vi "GNSS RF Test Set Parameters.vi"(8 "error in (no error)":errorcluster, 10 "Parameters":T1={"GNSS Standard"=enum."GPS", "Frequency (Hz)"=0.0, "Auto Level"=FALSE, "Power (dBm)"=0.0, "External Attenuation (dB)"=0.0, "Measurement Interval (s)"=1000.0, "Pattern"=enum."PN9", "Enable Averaging"=FALSE, "Type Of Averaging"=enum."MEAN", "Number of Averages"=0, "Waveform Name"="", "Enable Traces"=FALSE} {"External Attenuation (dB)" format="%.1g"; "Power (dBm)" format="%.1g"}, 11 "Template Tx Test in":refnum<class "niDTS GNSS RF Test.lvclass">) -> (0 "error out":errorcluster, 3 "Template Tx Test out":refnum<class "niDTS GNSS RF Test.lvclass">)   [LabVIEW 2015, in "niDTS GNSS.lvlib" / "niDTS GNSS RF Test.lvclass"]
uses:
  niDTS GNSS RF Test.lvclass
  Includes/niDTS GNSS RF Test INC Parameters.ctl
  niDTS GNSS RF Test.lvclass/niDTS GNSS RF Test.ctl
  niDTS GNSS.lvlib
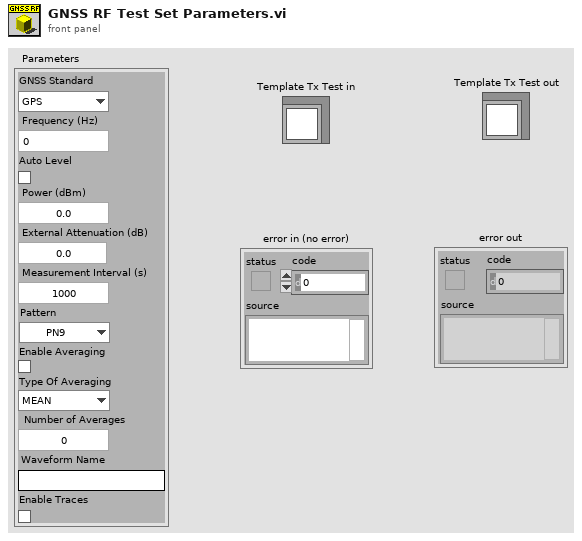
[diagram p1: front panel]
types:
  T1 = typedef "niDTS GNSS.lvlib/niDTS GNSS RF Test INC Parameters.ctl" = cluster{"GNSS Standard":enum16{"GPS", "GLONASS", "Galileo", "Beidou"}, "Frequency (Hz)":dbl, "Auto Level":bool, "Power (dBm)":dbl, "External Attenuation (dB)":dbl, "Measurement Interval (s)":dbl, "Pattern":enum16{"0", "1", "01", "00001111", "PN9"}, "Enable Averaging":bool, "Type Of Averaging":enum16{"MEAN", "MAX", "MIN", "MAXMIN"}, "Number of Averages":i32, "Waveform Name":string, "Enable Traces":bool}
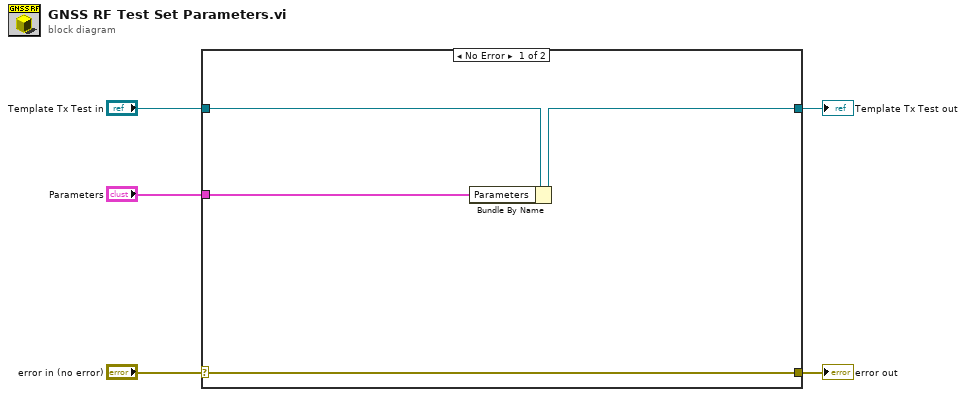
[diagram p0: block diagram]
diagram:
  n1 = case shown="No Error" "error in (no error)" {
    selector: "error in (no error)" -> [w9 w11]
    tunnel: [w9 w11] -> w4
    tunnel: [w7 w10] -> w2
    tunnel: "Template Tx Test in" -> [w8 w10]
    tunnel: "Parameters" -> [w6 _]
    frame No Error {
      n2 = Bundle By Name(cluster=w8, "Parameters"=w6) -> (w7:refnum<class "niDTS GNSS RF Test.lvclass">)
    }
    frame Error {
    }
  }
  "error out" <- w4
  "Template Tx Test out" <- w2
